vi "Receptor Fortu.vi"() -> ()   [LabVIEW 2020]
uses:
  <vilib>/Instr/_visa.llb/VISA Configure Serial Port (Instr).vi
panel:
  in  "String":string
  in  "stop":bool
  in  "VISA resource name":refnum<visa-resource-name>
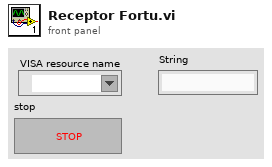
[diagram p1: front panel]
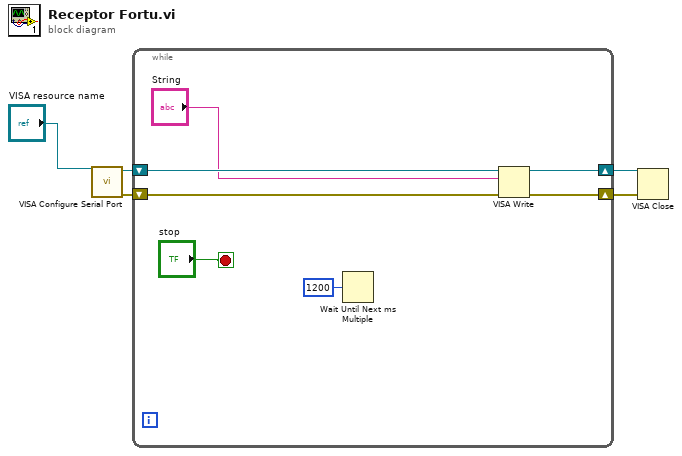
[diagram p0: block diagram]
diagram:
  n1 = call-poly "VISA Configure Serial Port"("VISA resource name"="VISA resource name") -> ("VISA resource name out"=w5:refnum<visa-resource-name>, "error out"=w4:errorcluster)  [unwired: 13 in]
  n2 = while {
    shift-right: [w11] -> w3
    shift-left: w5 -> [w8]
    shift-right: [w10] -> w2
    shift-left: w4 -> [w9]
    stop <- "stop" stop-if-true
    n3 = Wait Until Next ms Multiple(millisecond multiple=u32 1200) -> ()  [unwired: 1 out]
    n4 = VISA Write(VISA resource name=w8, write buffer="String", error in (no error)=w9) -> (VISA resource name out=w11:refnum<visa-resource-name>, error out=w10:errorcluster)  [unwired: 1 out]
  }
  n5 = VISA Close(VISA resource name=w3, error in (no error)=w2) -> ()  [unwired: 1 out]
